vi "TextMark_write.vi"(8 "error in (no error)":errorcluster, 11 "Stimulus parameters":T1) -> ()   [LabVIEW 2016]
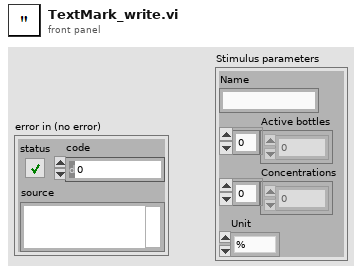
[diagram p1: front panel]
types:
  T1 = cluster{"Name":string, "Active bottles":i32[], "Concentrations":dbl[], "Unit":enum16{"%", "ppm"}}
  T2 = cluster{"VISA Refnum in":refnum<visa-resource-name>, "error in (no error)":errorcluster}
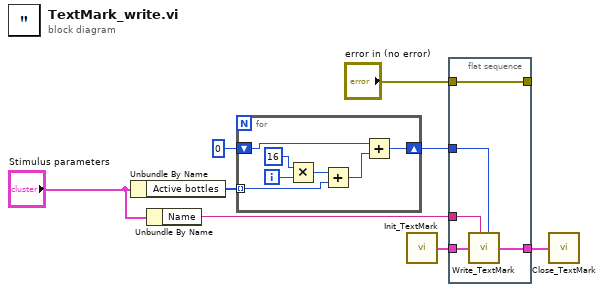
[diagram p0: block diagram]
diagram:
  n1 = Unbundle By Name("Stimulus parameters") -> ("Active bottles"=w3:i32[])
  n2 = Unbundle By Name("Stimulus parameters") -> ("Name"=w5:string)
  n3 = for {
    tunnel: w3 -> [w15] mode=indexing
    shift-right: [w9] -> w1
    shift-left: 0 -> [w11]
    i -> [w13]
    n4 = Multiply(x=16, y=w13) -> (x*y=w12:i32)
    n5 = Add(x=w12, y=w15) -> (x+y=w10:i32)
    n6 = Add(x=w11, y=w10) -> (x+y=w9:i32)
  }
  n7 = call "Init_TextMark.vi"() -> ("TextMark out"=w6:T2)
  n8 = flat-sequence {
    tunnel: w6 -> [w20]
    tunnel: [w19] -> w7
    tunnel: w5 -> [w18]
    tunnel: [w17] -> _
    tunnel: "error in (no error)" -> [w17]
    tunnel: w1 -> [w16]
    frame #0 {
      n9 = call "Write_TextMark.vi"("text"=w18, "TextMark in"=w20, "type"=w16) -> ("TextMark out"=w19:T2)  [unwired: 6 in]
    }
  }
  n10 = call "Close_TextMark.vi"("TextMark in"=w7) -> ()
